vi "Get Hi Low Times Dew Pt V.vi"(8 "error in (no error)":errorcluster, 10 "DateTimeLowDewPt":T1, 11 "DateTimeHiDewPt":T1) -> (0 "error out":errorcluster, 1 "function return":i16, 2 "DateTimeLowDewPt out":T1, 3 "DateTimeHiDewPt out":T1)   [LabVIEW 2009, in "VantagePro.lvlib"]
doc: "DllAccess short int _stdcall GetHiLowTimesDewPt_V (DateTime* DateTimeHiDewPt, DateTime* DateTimeLowDewPt);"
uses:
  VantagePro.lvlib
  <userlib>/VantagePro/VantagePro.dll
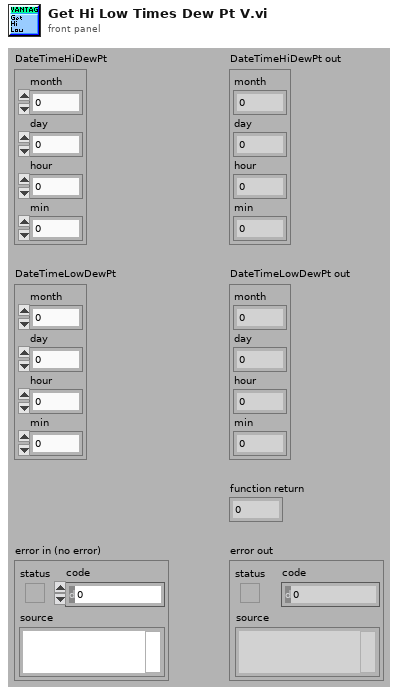
[diagram p1: front panel]
types:
  T1 = cluster{"month":i16, "day":i16, "hour":i16, "min":i16}
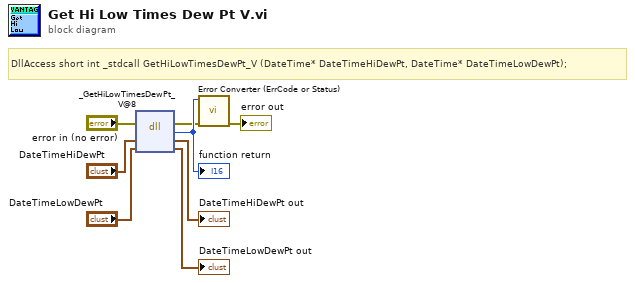
[diagram p0: block diagram]
diagram:
  # "DllAccess short int _stdcall GetHiLowTimesDewPt_V (DateTime* DateTimeHiDewPt, DateTime* DateTimeLowDewPt);"
  n1 = dll-call lib="C:/Program Files/National Instruments/LabVIEW 2010/user.lib/VantagePro/VantagePro.*" fn="_GetHiLowTimesDewPt_V@8"(error in="error in (no error)", "DateTimeHiDewPt"="DateTimeHiDewPt", "DateTimeLowDewPt"="DateTimeLowDewPt") -> (error out=w2:errorcluster, w8:i16, "DateTimeHiDewPt"=→"DateTimeHiDewPt out":T1, "DateTimeLowDewPt"=→"DateTimeLowDewPt out":T1)  [unwired: 2 in, 1 out]
  "function return" <- w8
  n2 = call "Error Converter (ErrCode or Status).vi"("error in (no error)"=w2, "error code"=w8) -> ("error out"=→"error out":errorcluster)  [unwired: 9 in]
